vi "Listener.vi"() -> ()   [LabVIEW 2015]
uses:
  ROS/Code/Console/Servers/ServerSubs/TopicDef.ctl
  ROS/Code/SubVIs/_ROSDirection.ctl
  ROS/MessageParsing/std_msgs/subs/parse_string_scalar.vi
panel:
  in  "Definitions":T1={"Topic"="/chatter", "Type"="std_msgs/String", "Action"=enum."Subscriber", "Update (ms)"=1, "queue size"=1}
  out "String":string
  in  "Stop Button":bool
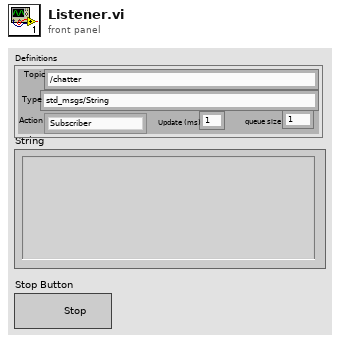
[diagram p1: front panel]
types:
  T1 = typedef "TopicDef.ctl" = cluster{"Topic":string, "Type":string, "Action":T2, "Update (ms)":u16, "queue size":u16}
  T2 = typedef "_ROSDirection.ctl" = enum16{"Node", "Publisher", "Subscriber", "ServiceClient", "ServiceProvider"}
  T3 = typedef "_ROSControl.ctl" = cluster{"topic port":u16, "Node":string, "topic":string, "type":string, "node port":u16, "error ":errorcluster, "Direction":T2, "Update (ms)":u16, "FIFO size":u16}
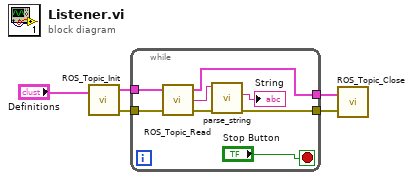
[diagram p0: block diagram]
diagram:
  n1 = call "ROS_Topic_Init.vi"("Definitions"="Definitions") -> ("ROS out"=w2:T3, "error out"=w1:errorcluster)  [unwired: 2 in]
  n2 = while {
    tunnel: [w12] -> w5
    tunnel: [w8] -> w4
    tunnel: w2 -> [w6]
    tunnel: w1 -> [w7]
    stop <- "Stop Button" stop-if-true
    n3 = call "ROS_Topic_Read.vi"("error in (no error)"=w7, "ROS in"=w6) -> ("error out"=w9:errorcluster, "Reply"=w10:string, "ROS out"=w12:T3)  [unwired: 1 in]
    n4 = call-poly "parse_string.vi"("error in"=w9, "msg in"=w10) -> ("error out"=w8:errorcluster, "string"=→"String":string)  [unwired: 3 in, 1 out]
  }
  n5 = call "ROS_Topic_Close.vi"("error in"=w4, "ROS in"=w5) -> ()  [unwired: 2 in, 1 out]
